vi "创建数组.vi"() -> ()   [LabVIEW 2020]
doc: "本VI是为《我和LabVIEW》一书编写的示例。\n关于本书的介绍请参考网页：\nhttp://ruanqizhen.spaces.live.com/blog/cns!5852D4F797C53FB6!4310.entry"
panel:
  out "添加一个元素":string[](array[string])
  out "变成一维数组":string[](array[string])
  out "默认变成二维数组":string[][](array[string])
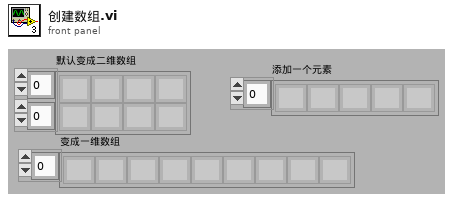
[diagram p1: front panel]
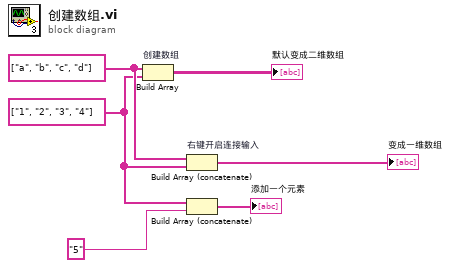
[diagram p0: block diagram]
diagram:
  w5 = string[] ["1", "2", "3", "4"] ("数组")
  w6 = string[] ["a", "b", "c", "d"] ("数组")
  n1 = Build Array "创建数组"(w6, w5) -> (→"默认变成二维数组":string[][])
  n2 = Build Array (concatenate) "右键开启连接输入"(w6, w5) -> (→"变成一维数组":string[])
  n3 = Build Array (concatenate)(w5, "5") -> (→"添加一个元素":string[])
